vi "fpga_main_fsm.vi"() -> ()   [LabVIEW 2019]
uses:
  fpga-aux/extern commands 3.ctl
  <vilib>/Platform/TimedLoop/XDataNode/timing_clust.ctl
  <vilib>/Platform/TimedLoop/XDataNode/nitl_modes.ctl
  <vilib>/Platform/TimedLoop/XDataNode/wakeup.ctl
  FPGA-Warsaw/Master FSM states.ctl
  <vilib>/rvi/Emulation/niFpgaGetClockAttributes.vi
  <vilib>/rvi/Emulation/niFpgaSctlEmulationGetInTimedLoop.vi
  <vilib>/rvi/Emulation/niFpgaEmulationReportErrorSimple.vi
  <vilib>/rvi/Emulation/niFpgaProcessEmulError.vi
  <vilib>/rvi/Emulation/niFpgaCriticalErrorInLSC.vi
  <vilib>/rvi/interface/RandomDataEmulation/niFpgaRandomDataHandleErrors.vi
  <vilib>/rvi/Memory/Memory_Emulation/nirvimemoryEmulation.vi
  <vilib>/rvi/Memory/Memory_Emulation/nirvimemoryFastEmulation.vi
  <vilib>/rvi/DataTransferAndStorage/Container/Common/niFpgaContainerGetUniqueNameForEmu.vi
  <vilib>/rvi/Memory/Memory_Emulation/niFpgaMemoryEmulationCacheClearOnFirstRun.vi
  <vilib>/rvi/Memory/Memory_Emulation/nirvimemoryEmulationManagerCache_MakeExclusive.vi
  <vilib>/rvi/Memory/Memory_Emulation/niFpgaMemoryEmulationValidateCache.vi
  <vilib>/rvi/Memory/Memory_Emulation/nirvimemoryEmulationManagerCache_InsertValue.vi
  <vilib>/Utility/error.llb/Clear Errors.vi
  <vilib>/rvi/Memory/Memory_Emulation/nirvimemoryEmulationManagerCache_ReleaseExclusive.vi
  <vilib>/rvi/Memory/Memory_Emulation/nirvimemoryEmulationManagerCache_GetValue.vi
  <vilib>/rvi/Emulation/niFpgaEmulationIsFPGAContextNoSignature.vi
  <vilib>/rvi/Memory/Memory_Emulation/nirvimemoryEmulationManagerCache_SetValue.vi
  <vilib>/rvi/Emulation/niFpgaSctlEmulationResourceMgr.vi
  <vilib>/rvi/eio/common/nirviEmuTemplateMethod_errors.vi
  <vilib>/rvi/DataTransferAndStorage/Container/XNode/niFpgaContainer.xnode
  <vilib>/rvi/interface/RandomDataEmulation/nirviRandomDataFpgaReadWriteTemplate.vi
  <vilib>/Platform/TimedLoop/XDataNode/XDataNode.xnode
  <vilib>/eio/EIONode/EIONode.xnode
  <vilib>/Platform/TimedLoop/XDataNode/XDNodeRunTimeDep.lvlib
panel:
  out "stall":bool=TRUE
  out "jmp":u32
  in  "stop":bool
  out "tim":u32
  out "extern cmmnd iter":i32 format="%.0x"
  out "prog data":u32
  out "wfm data":u32
  out "stall wait":i32 format="%.0x"
  out "extern command":T1
  out "aux (U24)":u32
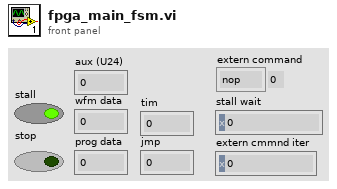
[diagram p1: front panel]
types:
  T1 = typedef "extern commands 3.ctl" = enum8{"nop", "dly", "wfm", "prog", "stop", "wait"}
  T2 = typedef "Master FSM states.ctl" = enum16{"reset", "0B", "1B", "2B", "wait", "trigwait"}
  T3 = cluster{"stall":bool, "NjumpT":u16, "PC":cluster{"PC":u16, "PC+1":u16}, "state":T2, "tim":u32, "wait":u32, "Njump":u16}
  T4 = typedef "XDNodeRunTimeDep.lvlib/timing_clust.ctl" = cluster{"Expected End [f-1]":u64, "Actual End [f-1]":u64, "Finished Late? [f-1]":bool, "Expected End [i-1]":u64, "Actual End [i-1]":u64, "Finished Late? [i-1]":bool, "Expected Start [i]":u64, "Actual Start [i]":u64, "Expected Start [f]":u64, "Actual Start [f]":u64, "Source Name":string, "Structure Name":string, "Period":i64, "Deadline":i64, "Offset":i64, "Start":i64, "Priority":i32, "Timeout":i32, "Mode":T5, "Wakeup Reason":T6, "Error":errorcluster, "Source Type":string, "Secondary Source Type":string, "Global End Time":u64, "Global Start Time":u64, "Frame Duration":u64, "Iteration Duration":u64, "Assigned CPU":i32, "I/O Scan Engine Mode":u32}
  T5 = typedef "XDNodeRunTimeDep.lvlib/nitl_modes.ctl" = enum32{"No Change", "Process missed periods, maintain original phase", "Discard missed periods, maintain original phase", "Process missed periods, ignore original phase", "Discard missed periods, ignore original phase"}
  T6 = typedef "XDNodeRunTimeDep.lvlib/wakeup.ctl" = enum32{"Normal", "Aborted", "Asynchronous wakeup", "Timing source error", "Timed loop error", "Timeout"}
  T7 = enum8{"jmp", "dly", "Con0 P0 out", "dds0 aux", "dds1 aux", "dds0 cmd", "dds1 cmd", "AOwfm", "AIacq", "rec ctl", "irq0", "dma point ", "stall", "dds2 aux", "dds3 aux", "dds2 cmd", "dds3 cmd", "trigwait", "jmp_X", "jmp_Y", "mcdA_init", "jmp_mcdA", "init_T", "jmp_T", "read_mcdA", "reset_jmp"}
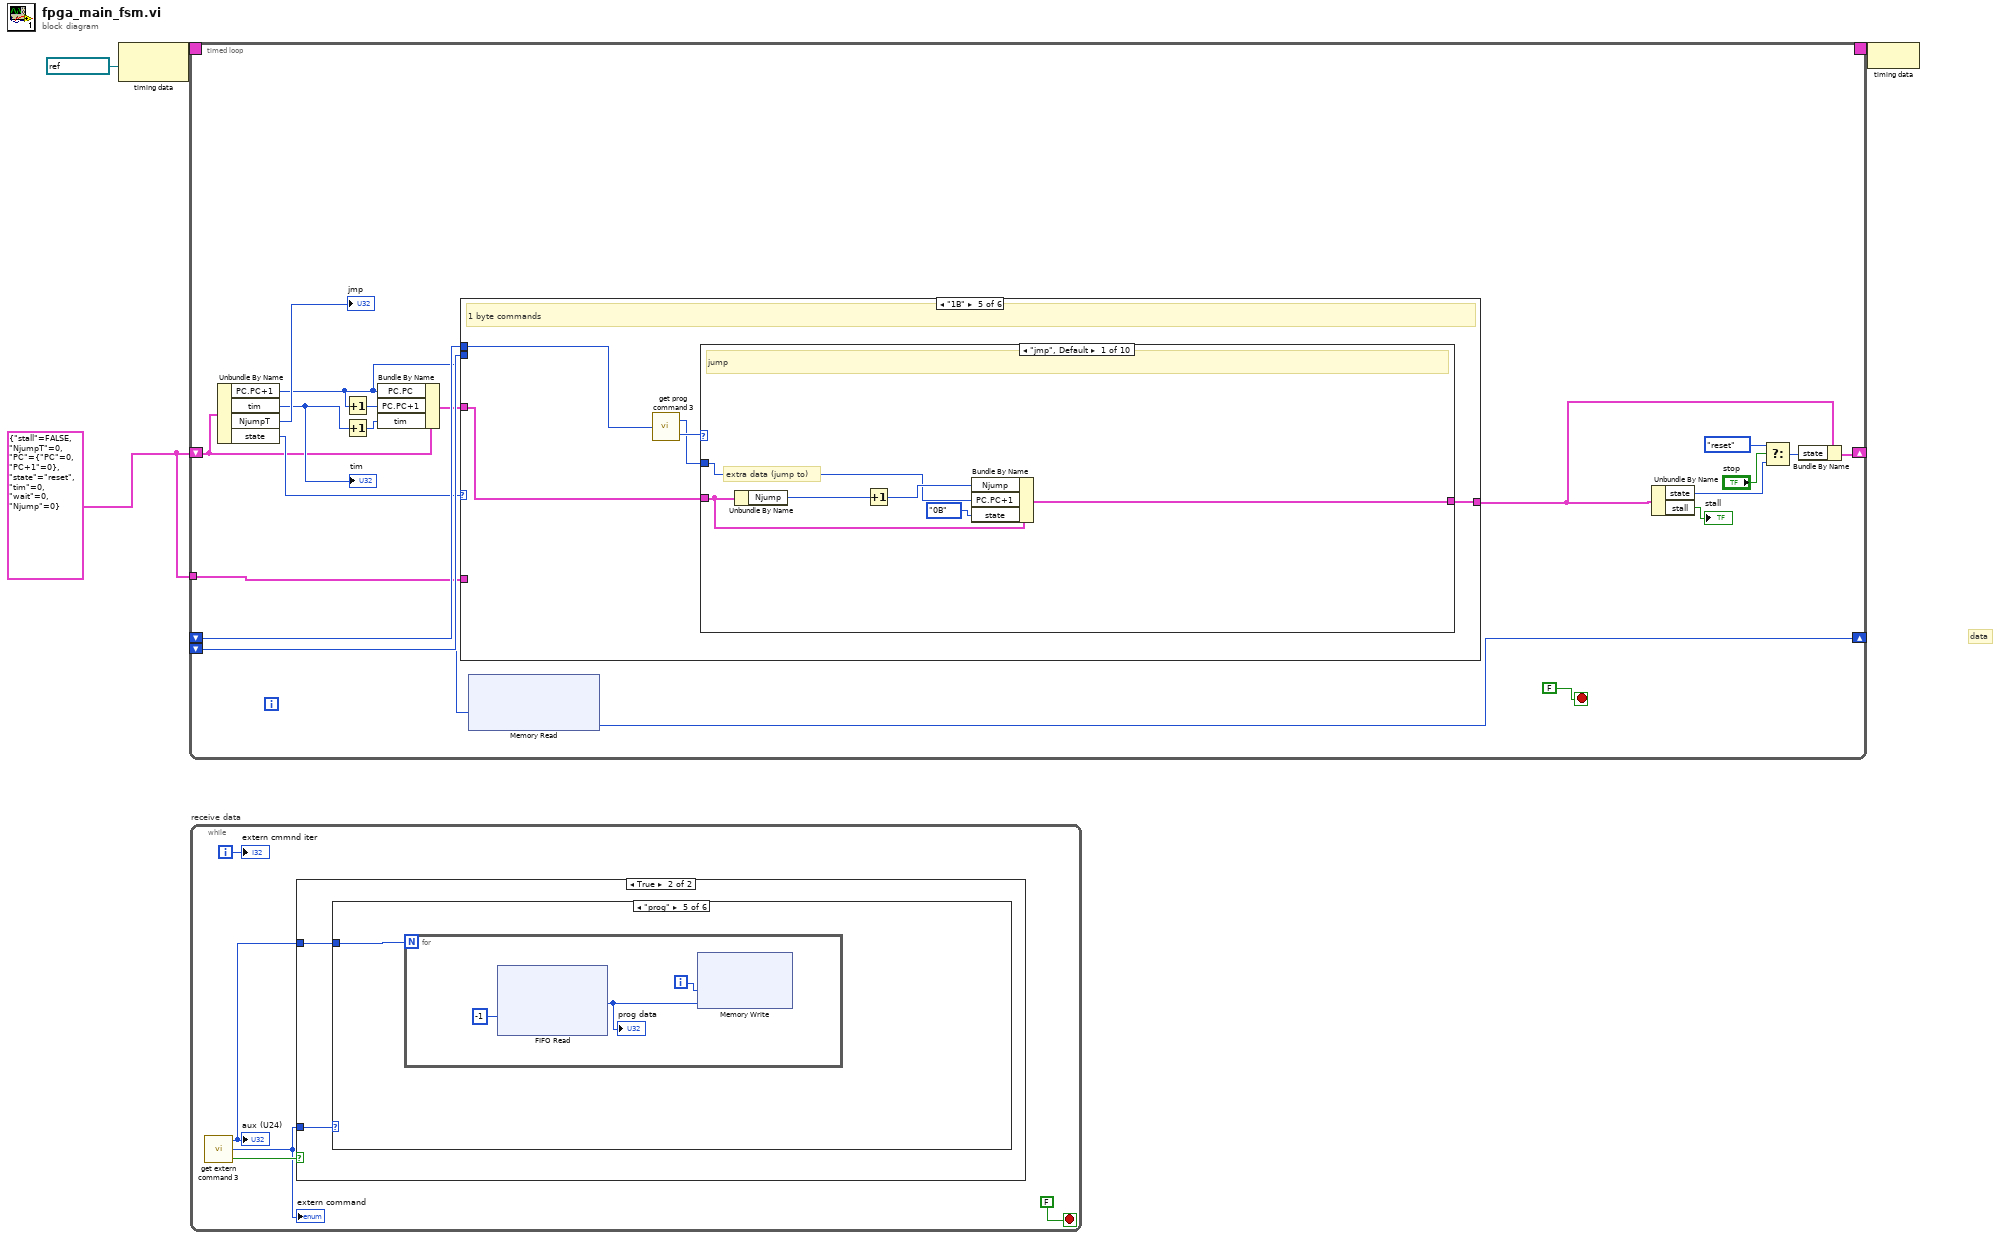
[diagram p0: block diagram]
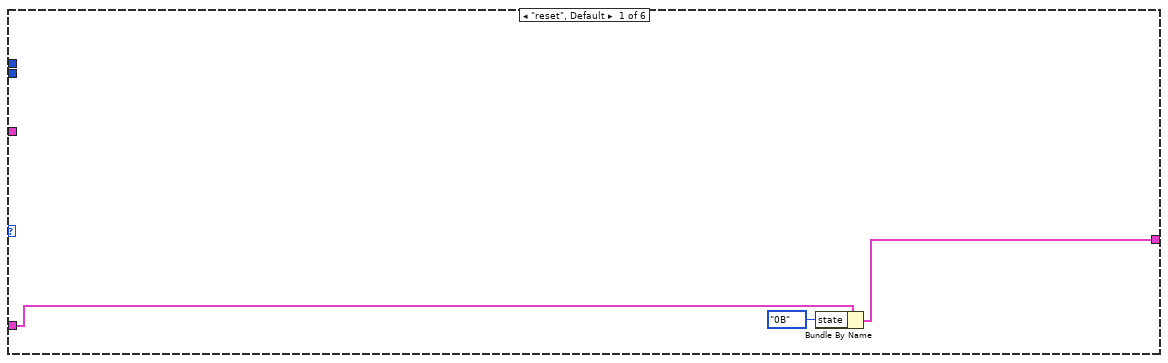
[diagram p2: hidden frame]
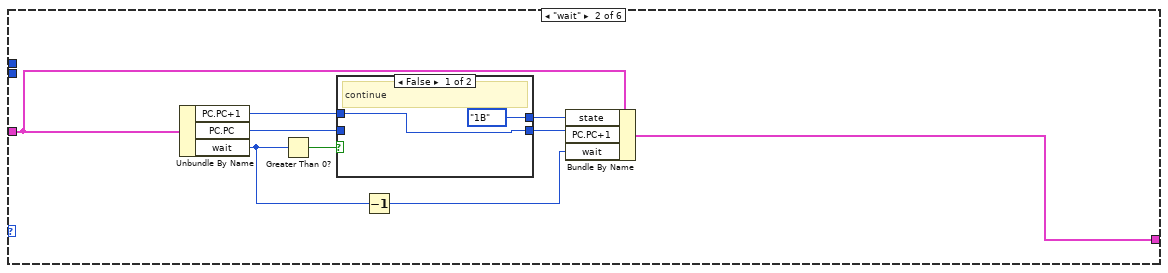
[diagram p3: hidden frame]
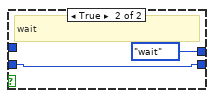
[diagram p4: hidden frame]
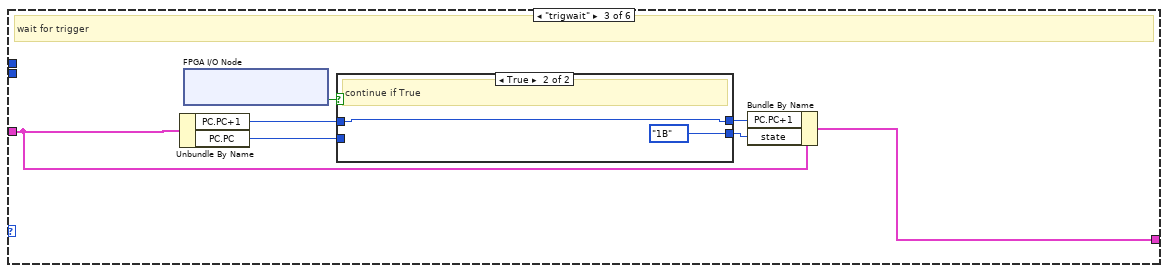
[diagram p5: hidden frame]
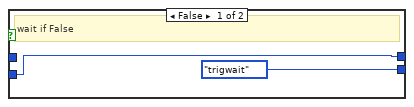
[diagram p6: hidden frame]
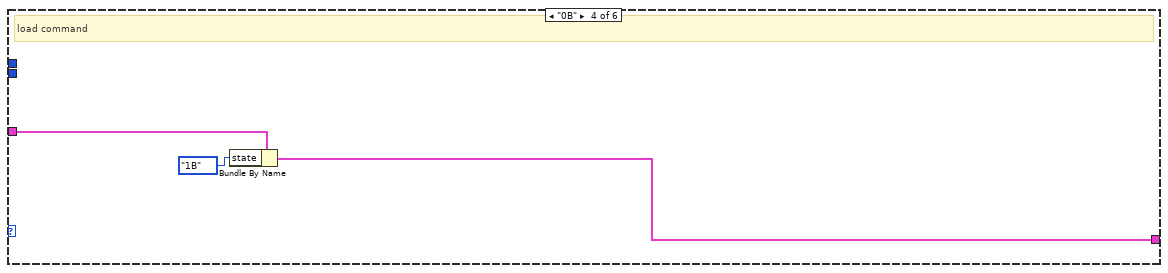
[diagram p7: hidden frame]
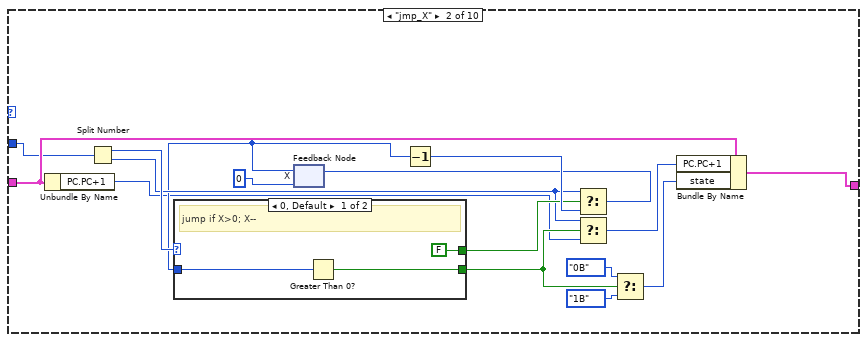
[diagram p8: hidden frame]
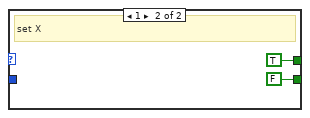
[diagram p9: hidden frame]
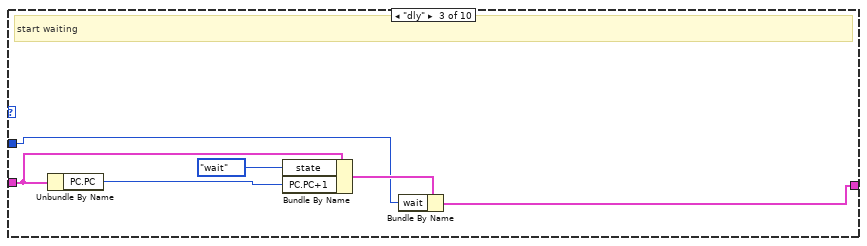
[diagram p10: hidden frame]
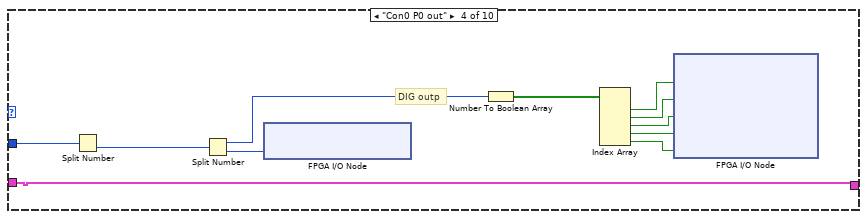
[diagram p11: hidden frame]
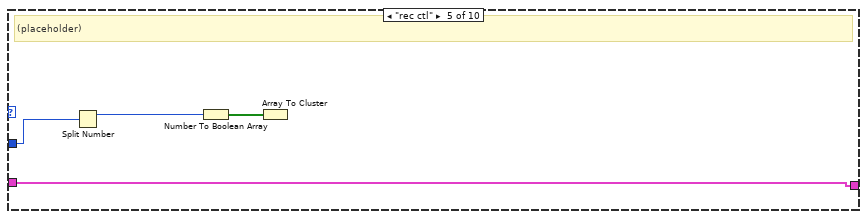
[diagram p12: hidden frame]
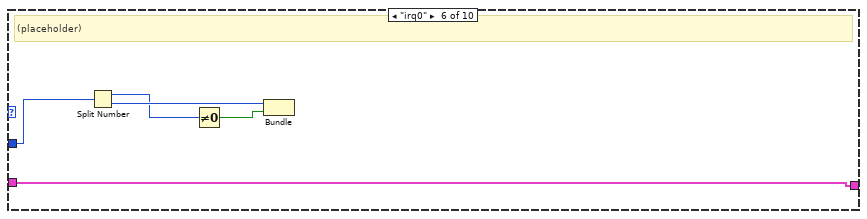
[diagram p13: hidden frame]
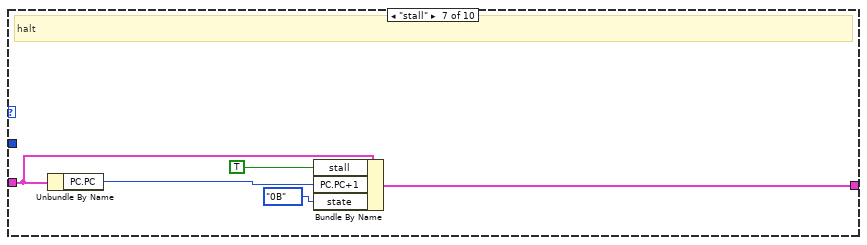
[diagram p14: hidden frame]
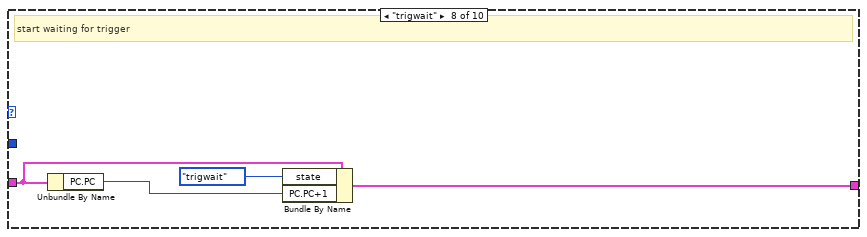
[diagram p15: hidden frame]
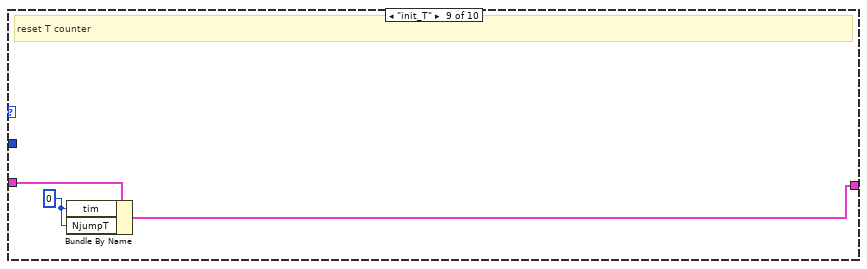
[diagram p16: hidden frame]
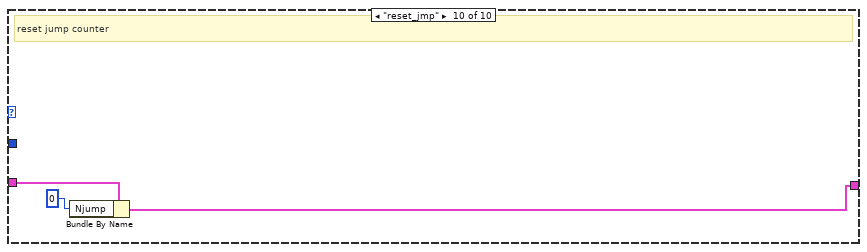
[diagram p17: hidden frame]
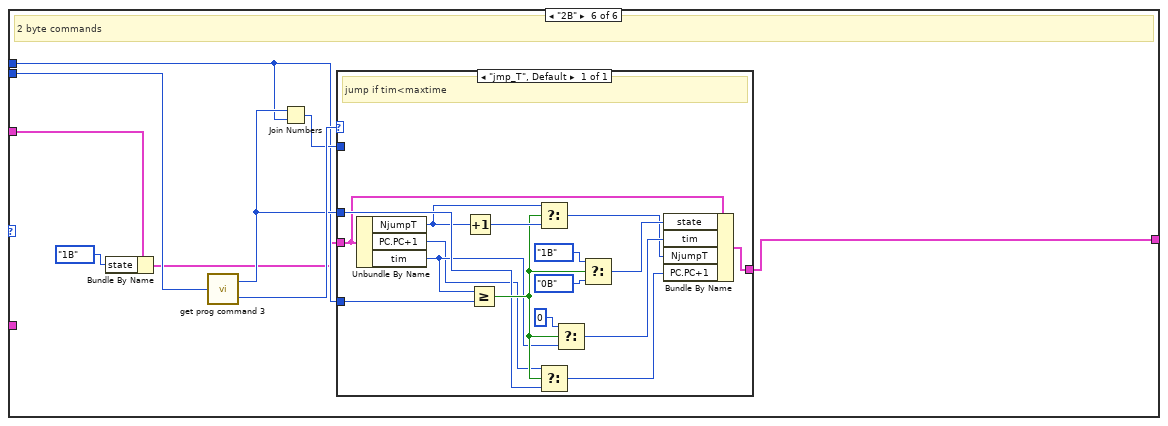
[diagram p18: hidden frame]
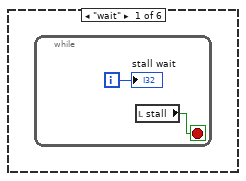
[diagram p20: hidden frame]
diagram:
  w1 = T3 {"stall"=FALSE, "NjumpT"=0, "PC"={"PC"=0, "PC+1"=0}, "state"=enum."reset", "tim"=0, "wait"=0, "Njump"=0} ("output cluster")
  # "data"
  n1 = node-c288(refnum<k21> "100MHz" ("Source Name")) -> (w4:T4)
  n2 = timed-loop {
    shift-right: [w24] -> _
    shift-left: _ -> [w23]
    shift-left: _ -> [w21]
    timing: w4 -> [_]
    timing-out: [_] -> w3
    shift-right: [w15] -> _
    shift-left: w1 -> [w6]
    tunnel: w1 -> [w8]
    stop <- FALSE stop-if-true
    n3 = Unbundle By Name(w6) -> ("PC.PC+1"=w5:u16, "tim"=w7:u32, "NjumpT"=→"jmp":u16, "state"=w11:T2)
    "tim" <- w7
    n4 = Increment(x=w5) -> (x+1=w19:u16)
    n5 = Increment(x=w7) -> (x+1=w20:u32)
    n6 = Bundle By Name(cluster=w6, "PC.PC"=w5, "PC.PC+1"=w19, "tim"=w20) -> (w9:T3)
    n7 = case shown="\"1B\"" w11 {
      tunnel: w23 -> [_ _ _ _ w59 w132]
      tunnel: w21 -> [_ _ _ _ _ w136]
      tunnel: w9 -> [_ w33 w44 w54 w58 w129]
      tunnel: [w26 w28 w41 w52 w55 w131] -> w14
      tunnel: w8 -> [w27 _ _ _ _ _]
      frame "reset", Default {
        n8 = Bundle By Name(cluster=w27, "state"=Master_FSM_states."0B") -> (w26:T3)
      }
      frame "wait" {
        n9 = Unbundle By Name(w33) -> ("PC.PC+1"=w32:u16, "PC.PC"=w31:u16, "wait"=w35:u32)
        n10 = Greater Than 0?(x=w35) -> (x > 0?=w36:bool)
        n11 = case shown="False" w36 {
          tunnel: w31 -> [_ w40]
          tunnel: w32 -> [w38 _]
          tunnel: [w38 w40] -> w30
          tunnel: [Master_FSM_states."1B" ("Enum") Master_FSM_states."wait" ("f")] -> w29
          frame False {
            # "continue"
          }
          frame True {
            # "wait"
          }
        }
        n12 = Decrement(x=w35) -> (x-1=w34:u32)
        n13 = Bundle By Name(cluster=w33, "state"=w29, "PC.PC+1"=w30, "wait"=w34) -> (w28:T3)
      }
      frame "trigwait" {
        # "wait for trigger"
        n14 = Unbundle By Name(w44) -> ("PC.PC+1"=w46:u16, "PC.PC"=w45:u16)
        n15 = xnode "FPGA I/O Node"() -> ("ConnectorA/DIO15"=w47:bool)  [unwired: 1 in, 1 out]
        n16 = case shown="True" w47 {
          tunnel: w45 -> [w49 _]
          tunnel: w46 -> [_ w51]
          tunnel: [w49 w51] -> w43
          tunnel: [Master_FSM_states."trigwait" ("f") Master_FSM_states."1B" ("Enum")] -> w42
          frame False {
            # "wait if False"
          }
          frame True {
            # "continue if True"
          }
        }
        n17 = Bundle By Name(cluster=w44, "PC.PC+1"=w43, "state"=w42) -> (w41:T3)
      }
      frame "0B" {
        # "load command"
        n18 = Bundle By Name(cluster=w54, "state"=Master_FSM_states."1B" ("Enum")) -> (w52:T3)
      }
      frame "1B" {
        # "1 byte commands"
        n19 = call "get prog command 3.vi"("Data"=w59) -> ("aux (24)"=w56:u32, "command"=w57:T7)
        n20 = case shown="\"jmp\", Default" w57 {
          tunnel: w58 -> [w63 w69 w92 w93 w104 w108 w115 w119 w124 w127]
          tunnel: [w64 w71 w88 w93 w104 w108 w117 w120 w123 w126] -> w55
          tunnel: w56 -> [w60 w67 w87 w94 w105 w109 _ _ _ _]
          frame "jmp", Default {
            # "extra data (jump to)"
            # "jump"
            n21 = Unbundle By Name(w63) -> ("Njump"=w65:u16)
            n22 = Increment(x=w65) -> (x+1=w62:u16)
            n23 = Bundle By Name(cluster=w63, "Njump"=w62, "PC.PC+1"=w60, "state"=Master_FSM_states."0B" ("Enum")) -> (w64:T3)
          }
          frame "jmp_X" {
            n24 = Unbundle By Name(w69) -> ("PC.PC+1"=w66:u16)
            n25 = Split Number(x=w67) -> (hi(x)=w77:u16, lo(x)=w75:u16)
            n26 = feedback #1 "X"(u16 0) -> (w74:u16)
            n27 = case shown="0, Default" w77 {
              tunnel: [FALSE ("s") TRUE ("s")] -> w76
              tunnel: w74 -> [w84 _]
              tunnel: [w83 FALSE] -> w73
              frame 0, Default {
                # "jump if X>0; X--"
                n28 = Greater Than 0?(x=w84) -> (x > 0?=w83:bool)
              }
              frame 1 {
                # "set X"
              }
            }
            n29 = Decrement(x=w74) -> (x-1=w79:u16)
            n30 = Select(t=w75, s=w76, f=w79) -> (s? t:f=w78:u16)
            n31 = feedback-in #1(w78) -> ()
            n32 = Select(t=w75, s=w73, f=w66) -> (s? t:f=w70:u16)
            n33 = Select(t=Master_FSM_states."0B" ("Enum"), s=w73, f=Master_FSM_states."1B" ("Enum")) -> (s? t:f=w72:T2)
            n34 = Bundle By Name(cluster=w69, "PC.PC+1"=w70, "state"=w72) -> (w71:T3)
          }
          frame "dly" {
            # "start waiting"
            n35 = Unbundle By Name(w92) -> ("PC.PC"=w90:u16)
            n36 = Bundle By Name(cluster=w92, "state"=Master_FSM_states."wait" ("Enum"), "PC.PC+1"=w90) -> (w89:T3)
            n37 = Bundle By Name(cluster=w89, "wait"=w87) -> (w88:T3)
          }
          frame "Con0 P0 out" {
            # "DIG outp"
            n38 = Split Number(x=w94) -> (lo(x)=w103:u16)  [unwired: 1 out]
            n39 = Split Number(x=w103) -> (hi(x)=w101:u8, lo(x)=w102:u8)
            n40 = xnode "FPGA I/O Node"("ConnectorA/DIO7:0"=w102) -> ()  [unwired: 1 in, 1 out]
            n41 = Number To Boolean Array(number=w101) -> (Boolean array=w100:bool[])
            n42 = Index Array(array=w100) -> (element #1=w99:bool, element #2=w98:bool, element #3=w97:bool, element #4=w96:bool, element #5=w95:bool)  [unwired: 5 in]
            n43 = xnode "FPGA I/O Node"("ConnectorA/DIO8"=w99, "ConnectorA/DIO9"=w98, "ConnectorA/DIO10"=w97, "ConnectorA/DIO11"=w96, "ConnectorA/DIO12"=w95) -> ()  [unwired: 5 in, 5 out]
          }
          frame "rec ctl" {
            # "(placeholder)"
            n44 = Split Number(x=w105) -> (hi(x)=w106:u16)  [unwired: 1 out]
            n45 = Number To Boolean Array(number=w106) -> (Boolean array=w107:bool[])
            n46 = Array To Cluster(array=w107) -> ()  [unwired: 1 out]
          }
          frame "irq0" {
            # "(placeholder)"
            n47 = Split Number(x=w109) -> (hi(x)=w111:u16, lo(x)=w112:u16)
            n48 = Not Equal To 0?(x=w111) -> (x != 0?=w110:bool)
            n49 = Bundle(w112, w110) -> ()  [unwired: 1 in, 1 out]
          }
          frame "stall" {
            # "halt"
            n50 = Unbundle By Name(w115) -> ("PC.PC"=w114:u16)
            n51 = Bundle By Name(cluster=w115, "stall"=TRUE ("stop"), "PC.PC+1"=w114, "state"=Master_FSM_states."0B") -> (w117:T3)
          }
          frame "trigwait" {
            # "start waiting for trigger"
            n52 = Unbundle By Name(w119) -> ("PC.PC"=w118:u16)
            n53 = Bundle By Name(cluster=w119, "state"=Master_FSM_states."trigwait" ("Enum"), "PC.PC+1"=w118) -> (w120:T3)
          }
          frame "init_T" {
            w122 = i16 0
            # "reset T counter"
            n54 = Bundle By Name(cluster=w124, "tim"=w122, "NjumpT"=w122) -> (w123:T3)
          }
          frame "reset_jmp" {
            # "reset jump counter"
            n55 = Bundle By Name(cluster=w127, "Njump"=u32 0 ("PC")) -> (w126:T3)
          }
        }
      }
      frame "2B" {
        # "2 byte commands"
        n56 = Bundle By Name(cluster=w129, "state"=Master_FSM_states."1B" ("Enum")) -> (w128:T3)
        n57 = call "get prog command 3.vi"("Data"=w136) -> ("aux (24)"=w134:u32, "command"=w135:T7)
        n58 = Join Numbers(hi=w134, lo=w132) -> ((hi.lo)=w133:u64)
        n59 = case shown="\"jmp_T\", Default" w135 {
          tunnel: w134 -> [w141]
          tunnel: w133 -> [_]
          tunnel: w132 -> [w142]
          tunnel: [w146] -> w131
          tunnel: w128 -> [w140]
          frame "jmp_T", Default {
            # "jump if tim<maxtime"
            n60 = Unbundle By Name(w140) -> ("NjumpT"=w139:u16, "PC.PC+1"=w137:u16, "tim"=w138:u32)
            n61 = Increment(x=w139) -> (x+1=w151:u16)
            n62 = Greater Or Equal?(x=w138, y=w142) -> (x >= y?=w150:bool)
            n63 = Select(t=w139, s=w150, f=w151) -> (s? t:f=w144:u16)
            n64 = Select(t=w137, s=w150, f=w141) -> (s? t:f=w143:u32)
            n65 = Select(t=u32 0 ("PC"), s=w150, f=w138) -> (s? t:f=w145:u32)
            n66 = Select(t=Master_FSM_states."1B" ("Enum"), s=w150, f=Master_FSM_states."0B" ("Enum")) -> (s? t:f=w147:T2)
            n67 = Bundle By Name(cluster=w140, "state"=w147, "tim"=w145, "NjumpT"=w144, "PC.PC+1"=w143) -> (w146:T3)
          }
        }
      }
    }
    n68 = xnode ("Memory Read")("Address"=w5) -> ("Data"=w24:u32)  [unwired: 1 in, 1 out]
    n69 = Unbundle By Name(w14) -> ("state"=w17:T2, "stall"=→"stall":bool)
    n70 = Select(t=Master_FSM_states."reset" ("Enum"), s="stop", f=w17) -> (s? t:f=w16:T2)
    n71 = Bundle By Name(cluster=w14, "state"=w16) -> (w15:T3)
  }
  n72 = while "receive data" {
    i -> [w158]
    stop <- FALSE stop-if-true
    n73 = call "get extern command 3.vi"() -> ("aux (U24)"=w156:u32, "extern command"=w155:T1, "valid command?"=w157:bool)  [unwired: 1 in]
    "extern command" <- w155
    "aux (U24)" <- w156
    n74 = case shown="True" w157 {
      tunnel: w155 -> [_ w161]
      tunnel: w156 -> [_ w160]
      frame False {
      }
      frame True {
        n75 = case shown="\"prog\"" w161 {
          tunnel: w160 -> [_ w164 w166 w167 w182 _]
          frame "wait" {
            n76 = while {
              i -> [w162]
              stop <- w163 stop-if-true
              n77 = local read "stall"() -> (w163:bool)
              "stall wait" <- w162
            }
          }
          frame "dly" {
            n78 = call "Wait"("Count(Ticks)"=w164) -> ()  [unwired: 1 out]
          }
          frame "stop" {
            n79 = Equal To 0?(x=w166) -> (x = 0?=w165:bool)
            n80 = local write "stop"(w165) -> ()
          }
          frame "wfm" {
            n81 = disable-structure shown="Disabled" {
              disable-tunnel: w167 -> [w171 _]
              frame Disabled {
                n82 = xnode ("FIFO Read")("Timeout"=-1) -> ("Element"=w169:u32)  [unwired: 1 in, 2 out]
                n83 = Split Number(x=w169) -> (lo(x)=w168:u16)  [unwired: 1 out]
                n84 = for {
                  N: w171 -> [_]
                  tunnel: w168 -> [w172]
                  i -> [w174]
                  n85 = Add(x=w174, y=w172) -> (x+y=w173:i32)
                  n86 = xnode ("FIFO Read")("Timeout"=-1) -> ("Element"=w176:u32)  [unwired: 1 in, 2 out]
                  "wfm data" <- w176
                  n87 = Logical Shift(y=1 ("x"), x=w173) -> (x << y=w178:i32)
                  n88 = Increment(x=w178) -> (x+1=w179:i32)
                  n89 = Split Number(x=w176) -> (hi(x)=w181:u16, lo(x)=w180:u16)
                  n90 = xnode ("Memory Write")("Address"=w179, "Data"=w180) -> ()  [unwired: 1 in, 1 out]
                  n91 = xnode ("Memory Write")("Address"=w178, "Data"=w181) -> ()  [unwired: 1 in, 1 out]
                }
              }
              frame Enabled {
              }
            }
          }
          frame "prog" {
            n92 = for {
              N: w182 -> [_]
              i -> [w183]
              n93 = xnode ("FIFO Read")("Timeout"=-1) -> ("Element"=w185:u32)  [unwired: 1 in, 2 out]
              "prog data" <- w185
              n94 = xnode ("Memory Write")("Address"=w183, "Data"=w185) -> ()  [unwired: 1 in, 1 out]
            }
          }
          frame "nop" {
          }
        }
      }
    }
    "extern cmmnd iter" <- w158
  }
  n95 = node-c288(w3) -> ()
